vi "Logout.vi"(8 "Error In":errorcluster, 11 "menu reference":refnum<k9>) -> (0 "Error Out":errorcluster)   [LabVIEW 2025, in "Full User Interface.lvlib"]
uses:
  Full User Interface.lvlib
  Localization/Section.ctl
  Localization/Localization.lvlib
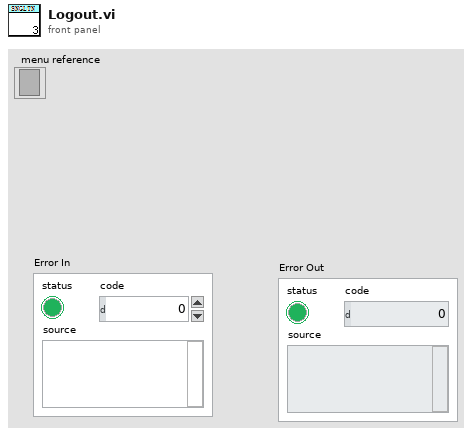
[diagram p1: front panel]
types:
  T1 = typedef "Localization.lvlib/Section.ctl" = enum16{"Menu", "Title", "Workstation Config"}
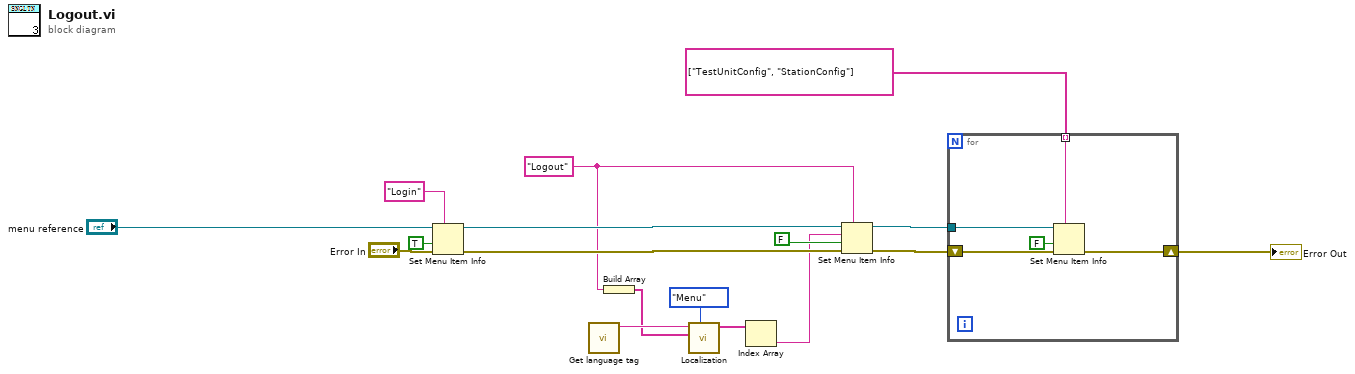
[diagram p0: block diagram]
diagram:
  w4 = "Logout"
  n1 = Set Menu Item Info(7:"Login", 8:"Error In", 9:TRUE ("enabled"), 11:"menu reference") -> (0:w13:errorcluster, 3:w14:refnum<k9>)  [unwired: 3 in]
  n2 = call "Get language tag.vi"() -> ("language tag"=w5:string)  [unwired: 11 in]
  n3 = Build Array(w4) -> (w3:string[])
  n4 = call "Localization.vi"("section"=Section."Menu", "key"=w3, "Language key"=w5) -> ("Value"=w2:string[])  [unwired: 7 in, 1 out]
  n5 = Index Array(array=w2) -> (element=w1:string)  [unwired: 1 in]
  n6 = Set Menu Item Info(7:w4, 8:w13, 9:FALSE ("enabled"), 10:w1, 11:w14) -> (0:w10:errorcluster, 3:w7:refnum<k9>)  [unwired: 2 in]
  n7 = for {
    shift-right: [w21] -> w9
    shift-left: w10 -> [w22]
    tunnel: string[] ["TestUnitConfig", "StationConfig"] ("item tags") -> [w20] mode=indexing
    tunnel: w7 -> [w19]
    n8 = Set Menu Item Info(7:w20, 8:w22, 9:FALSE ("enabled"), 11:w19) -> (0:w21:errorcluster)  [unwired: 3 in, 1 out]
  }
  "Error Out" <- w9
